vi "treat external command.vi"(8 "error in (no error)":errorcluster, 11 "Roda_Filtros in":refnum<class "Roda_Filtros.lvclass">) -> (0 "error out":errorcluster, 3 "Roda_Filtros out":refnum<class "Roda_Filtros.lvclass">)   [LabVIEW 2018, in "Roda_Filtros.lvclass"]
uses:
  Roda_Filtros.lvclass
  Roda_Filtros.lvclass/Roda_Filtros.ctl
  RxTx/RxTx.lvclass
panel:
  out "Filter":u16(ring) items=["Methane", "U", "B", "V", "R", "I", "Clear"]
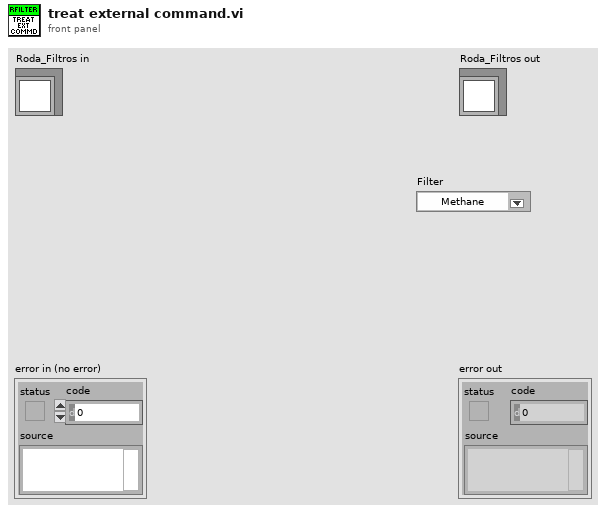
[diagram p1: front panel]
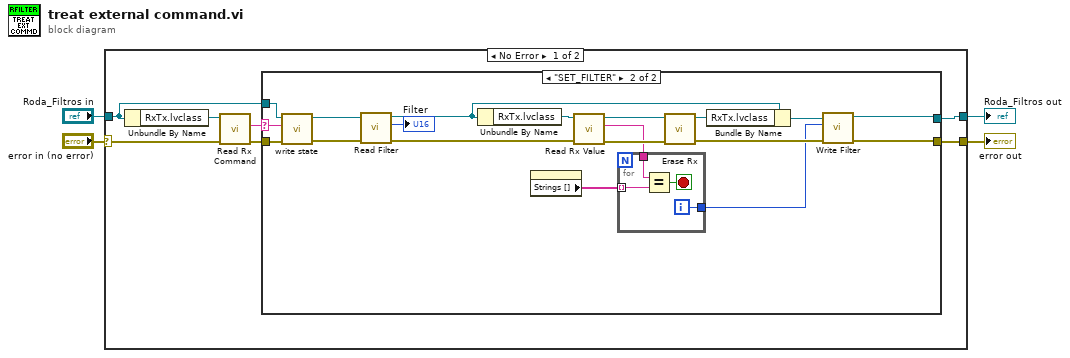
[diagram p0: block diagram]
diagram:
  n1 = case shown="No Error" "error in (no error)" {
    selector: "error in (no error)" -> [w10 w38]
    tunnel: [w6 w38] -> w3
    tunnel: [w8 w37] -> w1
    tunnel: "Roda_Filtros in" -> [w9 w37]
    frame No Error {
      n2 = Unbundle By Name(w9) -> ("RxTx.lvclass"=w11:refnum<class "RxTx.lvclass">)
      n3 = call "Read Rx Command.vi"("error in (no error)"=w10, "RxTx in"=w11) -> ("error out"=w7:errorcluster, "Rx Command"=w5:string)  [unwired: 7 in, 1 out]
      n4 = case shown="\"SET_FILTER\"" w5 {
        selector: w5 -> [_ w29]
        tunnel: w9 -> [w13 w32]
        tunnel: [w13 w17] -> w8
        tunnel: w7 -> [w12 w31]
        tunnel: [w12 w16] -> w6
        frame "False", Default {
        }
        frame "SET_FILTER" {
          n5 = call "write state.vi"("error in (no error)"=w31, "State"=w29, "Roda_Filtros in"=w32) -> ("error out"=w24:errorcluster, "Roda_Filtros out"=w25:refnum<class "Roda_Filtros.lvclass">)  [unwired: 7 in]
          n6 = call "Read Filter.vi"("error in (no error)"=w24, "Roda_Filtros in"=w25) -> ("error out"=w23:errorcluster, "Filter"=→"Filter":u16, "Roda_Filtros out"=w22:refnum<class "Roda_Filtros.lvclass">)  [unwired: 7 in]
          n7 = Unbundle By Name(w22) -> ("RxTx.lvclass"=w28:refnum<class "RxTx.lvclass">)
          n8 = property on="Filter" class="Ring (strict)"() -> ("Strings []"=w20:string[])  [unwired: 2 in, 2 out]
          n9 = call "Read Rx Value.vi"("error in (no error)"=w23, "RxTx in"=w28) -> ("error out"=w26:errorcluster, "Rx value"=w19:string, "RxTx out"=w27:refnum<class "RxTx.lvclass">)  [unwired: 7 in]
          n10 = for {
            tunnel: w20 -> [w36] mode=indexing
            tunnel: w19 -> [w35]
            tunnel: [w33] -> w14
            i -> [w33]
            stop <- w34 stop-if-true
            n11 = Equal?(x=w35, y=w36) -> (x = y?=w34:bool)
          }
          n12 = call "Erase Rx.vi"("error in (no error)"=w26, "RxTx in"=w27) -> ("error out"=w15:errorcluster, "RxTx out"=w30:refnum<class "RxTx.lvclass">)  [unwired: 8 in]
          n13 = Bundle By Name(cluster=w22, "RxTx.lvclass"=w30) -> (w18:refnum<class "Roda_Filtros.lvclass">)
          n14 = call "Write Filter.vi"("error in (no error)"=w15, "Filter"=w14, "Roda_Filtros in"=w18) -> ("error out"=w16:errorcluster, "Roda_Filtros out"=w17:refnum<class "Roda_Filtros.lvclass">)  [unwired: 7 in]
        }
      }
    }
    frame Error {
    }
  }
  "error out" <- w3
  "Roda_Filtros out" <- w1
